vi "new.uxx.be.vi"(0 "buffer (U64)":u64[](array[numeric])=[3026420053433122816, 0, 0, 0, 0, 0, 0, 0, 0] format="%016x", 1 "Start.Idx":u8, 2 "Length":u8, 3 "Big.Endian?":bool=TRUE) -> (7 "Uxx.be":u64 format="%.0x")   [LabVIEW 2022 SP3]
panel:
  out "U32.be 2":u32 format="%.0x"
  out "U8.be 2":u8 format="%.0x"
  out "U16.be 3":u16 format="%.0x"
  out "Mask 3":u64 format="%016x"
  out "U16.be 2":u16 format="%.0x"
  out "16bit integer":i16
  out "# of bytes to extract":u8
  out "Second Word.Shifted":u64 format="%016x"
  out "U32.be":u32 format="%.0x"
  out "Second Word":u64 format="%016x"
  out "Mask 2":u64 format="%016x"
  out "Mask":u64 format="%016x"
  out "# of already valid bytes":u8
  out "Left Shift (in bits)":u8
  out "Left Shift (in bytes)":u8
  out "First.Word":u64 format="%.0x"
  out "U8.be":u8 format="%.0x"
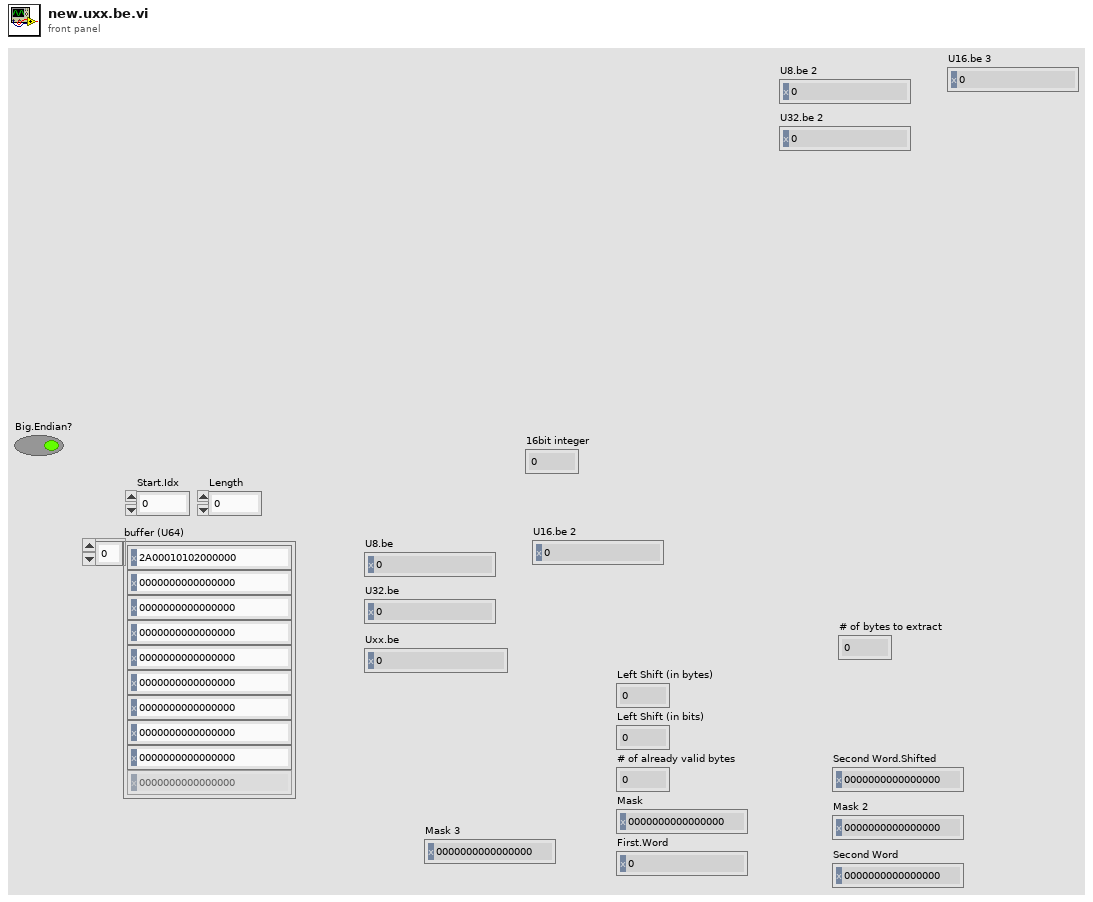
[diagram p1: front panel]
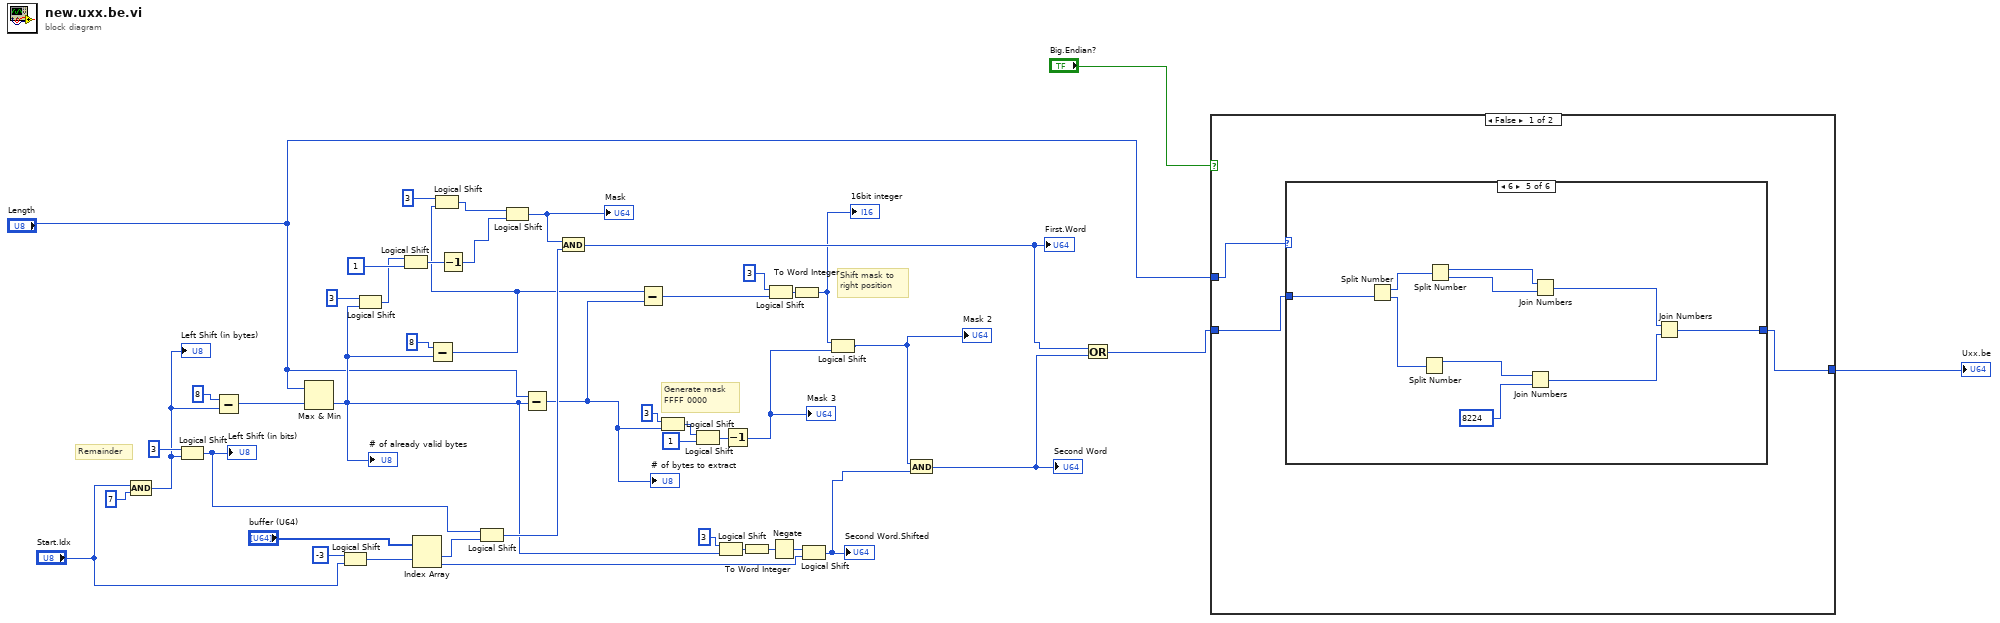
[diagram p0: block diagram]
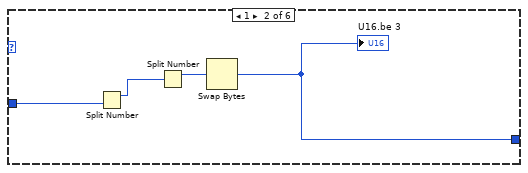
[diagram p3: hidden frame]
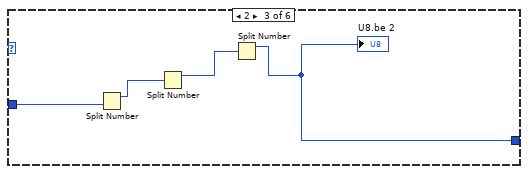
[diagram p4: hidden frame]
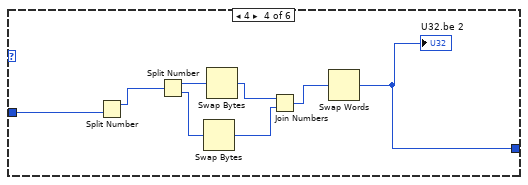
[diagram p5: hidden frame]
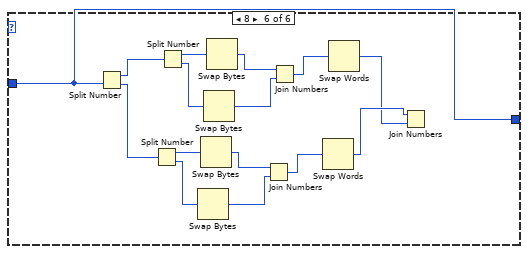
[diagram p6: hidden frame]
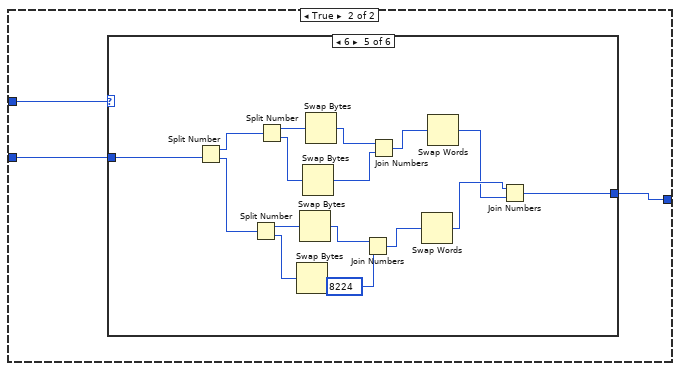
[diagram p7: hidden frame]
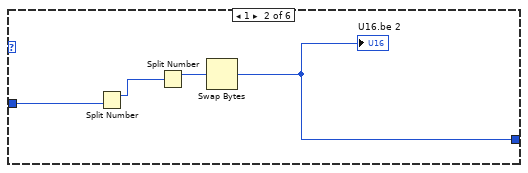
[diagram p9: hidden frame]
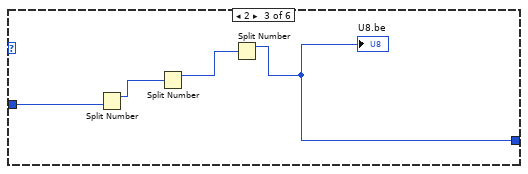
[diagram p10: hidden frame]
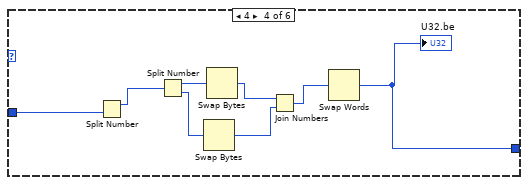
[diagram p11: hidden frame]
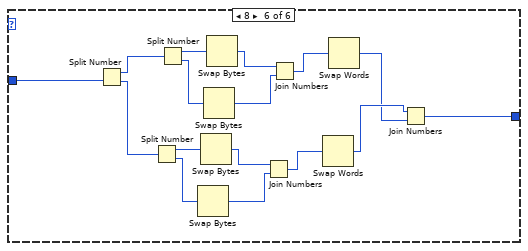
[diagram p12: hidden frame]
diagram:
  # "Remainder"
  # "Shift mask to\nright position"
  # "Generate mask\nFFFF 0000"
  n1 = And(x="Start.Idx", y=u8 7 ("x")) -> (x .and. y?=w36:u8)
  "Left Shift (in bytes)" <- w36
  n2 = Logical Shift(y=i16 3, x=w36) -> (x << y=w29:u8)
  "Left Shift (in bits)" <- w29
  n3 = Subtract(x=u8 8, y=w36) -> (x-y=w39:u8)
  n4 = Max & Min(x="Length", y=w39) -> (min(x,y)=w13:u8)  [unwired: 1 out]
  "# of already valid bytes" <- w13
  n5 = Logical Shift(y=i16 -3, x="Start.Idx") -> (x << y=w30:u8)
  n6 = Logical Shift(y=i16 3, x=w13) -> (x << y=w40:u8)
  n7 = Logical Shift(y=w40, x=u64 1) -> (x << y=w42:u64)
  n8 = Index Array(array="buffer (U64)", index #1=w30) -> (element #1=w28:u64, element #2=w22:u64)  [unwired: 1 in]
  n9 = Subtract(x=u8 8, y=w13) -> (x-y=w3:u8)
  n10 = Logical Shift(y=i16 3, x=w3) -> (x << y=w37:u8)
  n11 = Decrement(x=w42) -> (x-1=w35:u64)
  n12 = Logical Shift(y=w29, x=w28) -> (x << y=w26:u64)
  n13 = Logical Shift(y=w37, x=w35) -> (x << y=w27:u64)
  "Mask" <- w27
  n14 = Subtract(x="Length", y=w13) -> (x-y=w2:u8)
  "# of bytes to extract" <- w2
  n15 = And(x=w27, y=w26) -> (x .and. y?=w17:u64)
  "First.Word" <- w17
  n16 = Subtract(x=w3, y=w2) -> (x-y=w8:u8)
  n17 = Logical Shift(y=i16 3, x=w2) -> (x << y=w21:u8)
  n18 = Logical Shift(y=w21, x=u64 1) -> (x << y=w24:u64)
  n19 = Logical Shift(y=i16 3, x=w13) -> (x << y=w4:u8)
  n20 = Decrement(x=w24) -> (x-1=w9:u64)
  "Mask 3" <- w9
  n21 = To Word Integer(number=w4) -> (16bit integer=w6:i16)
  n22 = Logical Shift(y=i16 3, x=w8) -> (x << y=w19:u8)
  n23 = Negate(x=w6) -> (-x=w7:i16)
  n24 = To Word Integer(number=w19) -> (16bit integer=w15:i16)
  "16bit integer" <- w15
  n25 = Logical Shift(y=w7, x=w22) -> (x << y=w14:u64)
  "Second Word.Shifted" <- w14
  n26 = Logical Shift(y=w15, x=w9) -> (x << y=w12:u64)
  "Mask 2" <- w12
  n27 = And(x=w12, y=w14) -> (x .and. y?=w18:u64)
  "Second Word" <- w18
  n28 = Or(x=w17, y=w18) -> (x .or. y?=w16:u64)
  n29 = case shown="False" "Big.Endian?" {
    tunnel: w16 -> [w48 w93]
    tunnel: "Length" -> [w49 w92]
    tunnel: [w47 w91] -> w10
    frame False {
      n30 = case shown="6" w49 {
        tunnel: w48 -> [_ w51 w56 w63 w74 w76]
        tunnel: [_ w50 w54 w58 w71 w76] -> w47
        frame 0, Default {
        }
        frame 1 {
          n31 = Split Number(x=w51) -> (hi(x)=w53:u32)  [unwired: 1 out]
          n32 = Split Number(x=w53) -> (hi(x)=w52:u16)  [unwired: 1 out]
          n33 = Swap Bytes(anything=w52) -> (byte swapped=w50:u16)
          "U16.be 3" <- w50
        }
        frame 2 {
          n34 = Split Number(x=w56) -> (hi(x)=w57:u32)  [unwired: 1 out]
          n35 = Split Number(x=w57) -> (hi(x)=w55:u16)  [unwired: 1 out]
          n36 = Split Number(x=w55) -> (hi(x)=w54:u8)  [unwired: 1 out]
          "U8.be 2" <- w54
        }
        frame 4 {
          n37 = Split Number(x=w63) -> (hi(x)=w65:u32)  [unwired: 1 out]
          n38 = Split Number(x=w65) -> (hi(x)=w64:u16, lo(x)=w62:u16)
          n39 = Swap Bytes(anything=w62) -> (byte swapped=w59:u16)
          n40 = Swap Bytes(anything=w64) -> (byte swapped=w60:u16)
          n41 = Join Numbers(hi=w60, lo=w59) -> ((hi.lo)=w61:u32)
          n42 = Swap Words(1:w61) -> (0:w58:u32)
          "U32.be 2" <- w58
        }
        frame 6 {
          n43 = Split Number(x=w74) -> (hi(x)=w75:u32, lo(x)=w70:u32)
          n44 = Split Number(x=w70) -> (hi(x)=w72:u16)  [unwired: 1 out]
          n45 = Split Number(x=w75) -> (hi(x)=w68:u16, lo(x)=w73:u16)
          n46 = Join Numbers(hi=w72, lo=u16 8224 ("hi")) -> ((hi.lo)=w67:u32)
          n47 = Join Numbers(hi=w68, lo=w73) -> ((hi.lo)=w69:u32)
          n48 = Join Numbers(hi=w69, lo=w67) -> ((hi.lo)=w71:u64)
        }
        frame 8 {
          n49 = Split Number(x=w76) -> (hi(x)=w90:u32, lo(x)=w79:u32)
          n50 = Split Number(x=w79) -> (hi(x)=w84:u16, lo(x)=w83:u16)
          n51 = Split Number(x=w90) -> (hi(x)=w89:u16, lo(x)=w88:u16)
          n52 = Swap Bytes(anything=w83) -> (byte swapped=w80:u16)
          n53 = Swap Bytes(anything=w84) -> (byte swapped=w81:u16)
          n54 = Swap Bytes(anything=w88) -> (byte swapped=w85:u16)
          n55 = Swap Bytes(anything=w89) -> (byte swapped=w86:u16)
          n56 = Join Numbers(hi=w81, lo=w80) -> ((hi.lo)=w82:u32)
          n57 = Join Numbers(hi=w86, lo=w85) -> ((hi.lo)=w87:u32)
          n58 = Swap Words(1:w82) -> (0:w78:u32)
          n59 = Swap Words(1:w87) -> (0:w77:u32)
          n60 = Join Numbers(hi=w78, lo=w77) -> ()  [unwired: 1 out]
        }
      }
    }
    frame True {
      n61 = case shown="6" w92 {
        tunnel: w93 -> [_ w95 w100 w107 w123 w139]
        tunnel: [_ w94 w98 w102 w112 w126] -> w91
        frame 0, Default {
        }
        frame 1 {
          n62 = Split Number(x=w95) -> (hi(x)=w97:u32)  [unwired: 1 out]
          n63 = Split Number(x=w97) -> (hi(x)=w96:u16)  [unwired: 1 out]
          n64 = Swap Bytes(anything=w96) -> (byte swapped=w94:u16)
          "U16.be 2" <- w94
        }
        frame 2 {
          n65 = Split Number(x=w100) -> (hi(x)=w101:u32)  [unwired: 1 out]
          n66 = Split Number(x=w101) -> (hi(x)=w99:u16)  [unwired: 1 out]
          n67 = Split Number(x=w99) -> (hi(x)=w98:u8)  [unwired: 1 out]
          "U8.be" <- w98
        }
        frame 4 {
          n68 = Split Number(x=w107) -> (hi(x)=w109:u32)  [unwired: 1 out]
          n69 = Split Number(x=w109) -> (hi(x)=w108:u16, lo(x)=w106:u16)
          n70 = Swap Bytes(anything=w106) -> (byte swapped=w103:u16)
          n71 = Swap Bytes(anything=w108) -> (byte swapped=w104:u16)
          n72 = Join Numbers(hi=w104, lo=w103) -> ((hi.lo)=w105:u32)
          n73 = Swap Words(1:w105) -> (0:w102:u32)
          "U32.be" <- w102
        }
        frame 6 {
          n74 = Split Number(x=w123) -> (hi(x)=w125:u32, lo(x)=w115:u32)
          n75 = Split Number(x=w115) -> (hi(x)=w118:u16, lo(x)=w117:u16)
          n76 = Split Number(x=w125) -> (hi(x)=w124:u16, lo(x)=w122:u16)
          n77 = Swap Bytes(anything=w117) -> ()  [unwired: 1 out]
          n78 = Swap Bytes(anything=w118) -> (byte swapped=w111:u16)
          n79 = Swap Bytes(anything=w122) -> (byte swapped=w119:u16)
          n80 = Swap Bytes(anything=w124) -> (byte swapped=w120:u16)
          n81 = Join Numbers(hi=w111, lo=u16 8224 ("hi")) -> ((hi.lo)=w116:u32)
          n82 = Join Numbers(hi=w120, lo=w119) -> ((hi.lo)=w121:u32)
          n83 = Swap Words(1:w116) -> (0:w114:u32)
          n84 = Swap Words(1:w121) -> (0:w113:u32)
          n85 = Join Numbers(hi=w114, lo=w113) -> ((hi.lo)=w112:u64)
        }
        frame 8 {
          n86 = Split Number(x=w139) -> (hi(x)=w141:u32, lo(x)=w129:u32)
          n87 = Split Number(x=w129) -> (hi(x)=w134:u16, lo(x)=w133:u16)
          n88 = Split Number(x=w141) -> (hi(x)=w140:u16, lo(x)=w138:u16)
          n89 = Swap Bytes(anything=w133) -> (byte swapped=w130:u16)
          n90 = Swap Bytes(anything=w134) -> (byte swapped=w131:u16)
          n91 = Swap Bytes(anything=w138) -> (byte swapped=w135:u16)
          n92 = Swap Bytes(anything=w140) -> (byte swapped=w136:u16)
          n93 = Join Numbers(hi=w131, lo=w130) -> ((hi.lo)=w132:u32)
          n94 = Join Numbers(hi=w136, lo=w135) -> ((hi.lo)=w137:u32)
          n95 = Swap Words(1:w132) -> (0:w128:u32)
          n96 = Swap Words(1:w137) -> (0:w127:u32)
          n97 = Join Numbers(hi=w128, lo=w127) -> ((hi.lo)=w126:u64)
        }
      }
    }
  }
  "Uxx.be" <- w10
